vi "Generate ROI.vi"(5 "Rotate":dbl, 6 "Cluster":cluster{"上下边缘设置：":i32, "右边缘设置：":i32}, 7 "Centre":dbl[][](array[numeric]), 8 "error in (no error)":errorcluster, 10 "Command":enum16{"Top", "Bottom"}(ring), 11 "Image":T1) -> (0 "error out":errorcluster, 3 "Image Out":T1)   [LabVIEW 2016]
uses:
  <vilib>/vision/Image Controls.llb/IMAQ Image.ctl
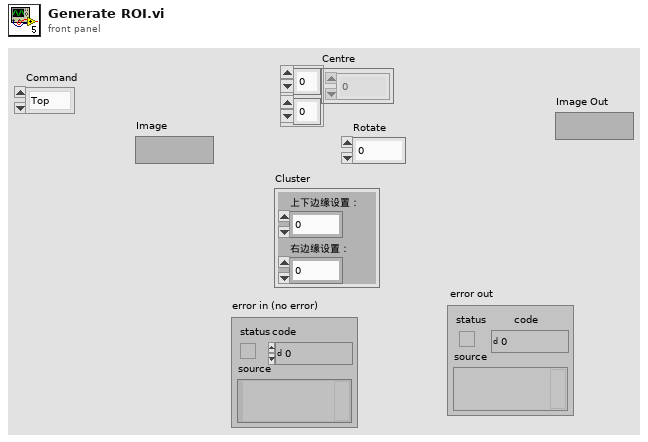
[diagram p1: front panel]
types:
  T1 = typedef "IMAQ Image.ctl" = refnum<image>
  T2 = typedef "IMAQ Rectangle" = cluster{"Left":i32, "Top":i32, "Right":i32, "Bottom":i32, "Rotation":dbl}
  T3 = typedef "ROI Descriptor" = cluster{"Global Rectangle":i32[], "Contours":cluster{"ID":enum32{"External", "Internal"}, "Type":u32, "Coordinates":i32[]}[]}
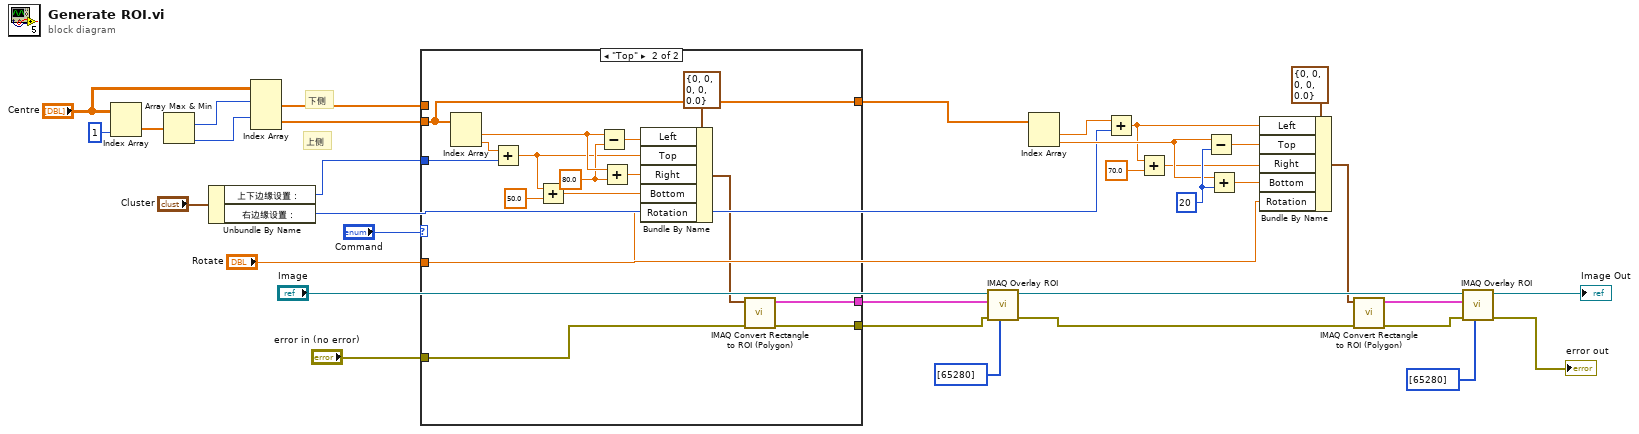
[diagram p0: block diagram]
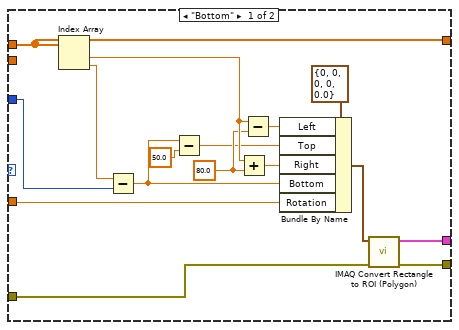
[diagram p2: hidden frame]
diagram:
  w12 = 20
  # "上侧"
  # "下侧"
  n1 = Index Array(array="Centre", index (col)=1 ("禁用的索引 (列)")) -> (element=w29:dbl[])  [unwired: 1 in]
  n2 = Array Max & Min(array=w29) -> (max index (indices)=w27:i32, min index (indices)=w26:i32)  [unwired: 2 out]
  n3 = Unbundle By Name("Cluster") -> ("上下边缘设置："=w24:i32, "右边缘设置："=w9:i32)
  n4 = Index Array(array="Centre", index (row) #1=w27, index (row) #2=w26) -> (element #1=w2:dbl[], element #2=w16:dbl[])  [unwired: 2 in]
  n5 = case shown="\"Top\"" "Command" {
    tunnel: [w48 w67] -> w35
    tunnel: [w49 w66] -> w34
    tunnel: "error in (no error)" -> [w50 w63]
    tunnel: w24 -> [w39 w57]
    tunnel: w16 -> [_ w52]
    tunnel: "Rotate" -> [w46 w53]
    tunnel: [w51 w52] -> w3
    tunnel: w2 -> [w51 _]
    frame "Bottom" {
      w43 = 80.0 ("y")
      n6 = Index Array(array=w51) -> (element #1=w44:dbl, element #2=w40:dbl)  [unwired: 2 in]
      n7 = Subtract(x=w40, y=w39) -> (x-y=w38:dbl)
      n8 = Subtract(x=w38, y=50.0) -> (x-y=w36:dbl)
      n9 = Add(x=w44, y=w43) -> (x+y=w41:dbl)
      n10 = Subtract(x=w44, y=w43) -> (x-y=w42:dbl)
      n11 = Bundle By Name(cluster=T2 {"Left"=0, "Top"=0, "Right"=0, "Bottom"=0, "Rotation"=0.0} ("Rectangle"), "Left"=w42, "Top"=w36, "Right"=w41, "Bottom"=w38, "Rotation"=w46) -> (w45:T2)
      n12 = call "IMAQ Convert Rectangle to ROI (Polygon)"("error in (no error)"=w50, "Rectangle"=w45) -> ("error out"=w49:errorcluster, "ROI Descriptor"=w48:T3)  [unwired: 6 in, 1 out]
    }
    frame "Top" {
      w59 = 80.0 ("y")
      n13 = Index Array(array=w52) -> (element #1=w60:dbl, element #2=w58:dbl)  [unwired: 2 in]
      n14 = Add(x=w58, y=w57) -> (x+y=w55:dbl)
      n15 = Add(x=w55, y=50.0) -> (x+y=w56:dbl)
      n16 = Subtract(x=w60, y=w59) -> (x-y=w62:dbl)
      n17 = Add(x=w60, y=w59) -> (x+y=w61:dbl)
      n18 = Bundle By Name(cluster=T2 {"Left"=0, "Top"=0, "Right"=0, "Bottom"=0, "Rotation"=0.0} ("Rectangle"), "Left"=w62, "Top"=w55, "Right"=w61, "Bottom"=w56, "Rotation"=w53) -> (w64:T2)
      n19 = call "IMAQ Convert Rectangle to ROI (Polygon)"("error in (no error)"=w63, "Rectangle"=w64) -> ("error out"=w66:errorcluster, "ROI Descriptor"=w67:T3)  [unwired: 6 in, 1 out]
    }
  }
  n20 = call "IMAQ Overlay ROI"("Colors (Green)"=u32[] [65280], "error in (no error)"=w34, "ROI Descriptor"=w35, "Image"="Image") -> ("error out"=w20:errorcluster, "Image Out"=w19:T1)  [unwired: 6 in]
  n21 = Index Array(array=w3) -> (element #1=w10:dbl, element #2=w11:dbl)  [unwired: 2 in]
  n22 = Add(x=w10, y=w9) -> (x+y=w8:dbl)
  n23 = Add(x=w8, y=70.0) -> (x+y=w6:dbl)
  n24 = Subtract(x=w11, y=w12) -> (x-y=w14:dbl)
  n25 = Add(x=w11, y=w12) -> (x+y=w13:dbl)
  n26 = Bundle By Name(cluster=T2 {"Left"=0, "Top"=0, "Right"=0, "Bottom"=0, "Rotation"=0.0} ("Rectangle"), "Left"=w8, "Top"=w14, "Right"=w6, "Bottom"=w13, "Rotation"="Rotate") -> (w17:T2)
  n27 = call "IMAQ Convert Rectangle to ROI (Polygon)"("error in (no error)"=w20, "Rectangle"=w17) -> ("error out"=w22:errorcluster, "ROI Descriptor"=w21:T3)  [unwired: 6 in, 1 out]
  n28 = call "IMAQ Overlay ROI"("Colors (Green)"=u32[] [65280], "error in (no error)"=w22, "ROI Descriptor"=w21, "Image"=w19) -> ("error out"=→"error out":errorcluster, "Image Out"=→"Image Out":T1)  [unwired: 6 in]
